vi "ADI_IMU_ADIS16448_AHRS_Madgwick2020.vi"(6 "Yaw Axis":enum16{"X", "Y", "Z"}(ring)=enum."Z", 8 "Reset?":bool, 9 "delta t":dbl, 11 "Data 2":T1) -> (3 "Output":cluster{"Pitch":dbl, "Roll":dbl, "Yaw":dbl})   [LabVIEW 2019]
panel:
  out "Quaternion":dbl[](array[numeric])
  in  "Beta":dbl=0.4
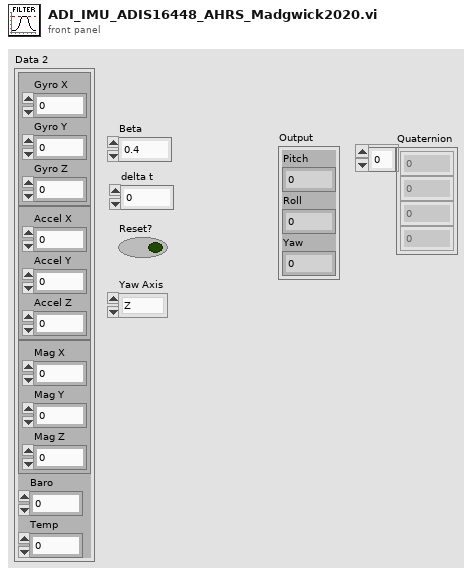
[diagram p1: front panel]
types:
  T1 = cluster{cluster{"Gyro X":dbl, "Gyro Y":dbl, "Gyro Z":dbl}, cluster{"Accel X":dbl, "Accel Y":dbl, "Accel Z":dbl}, cluster{"Mag X":dbl, "Mag Y":dbl, "Mag Z":dbl}, "Baro":dbl, "Temp":dbl}
  T2 = cluster{"Gyro X":dbl, "Gyro Y":dbl, "Gyro Z":dbl}
  T3 = cluster{"Accel X":dbl, "Accel Y":dbl, "Accel Z":dbl}
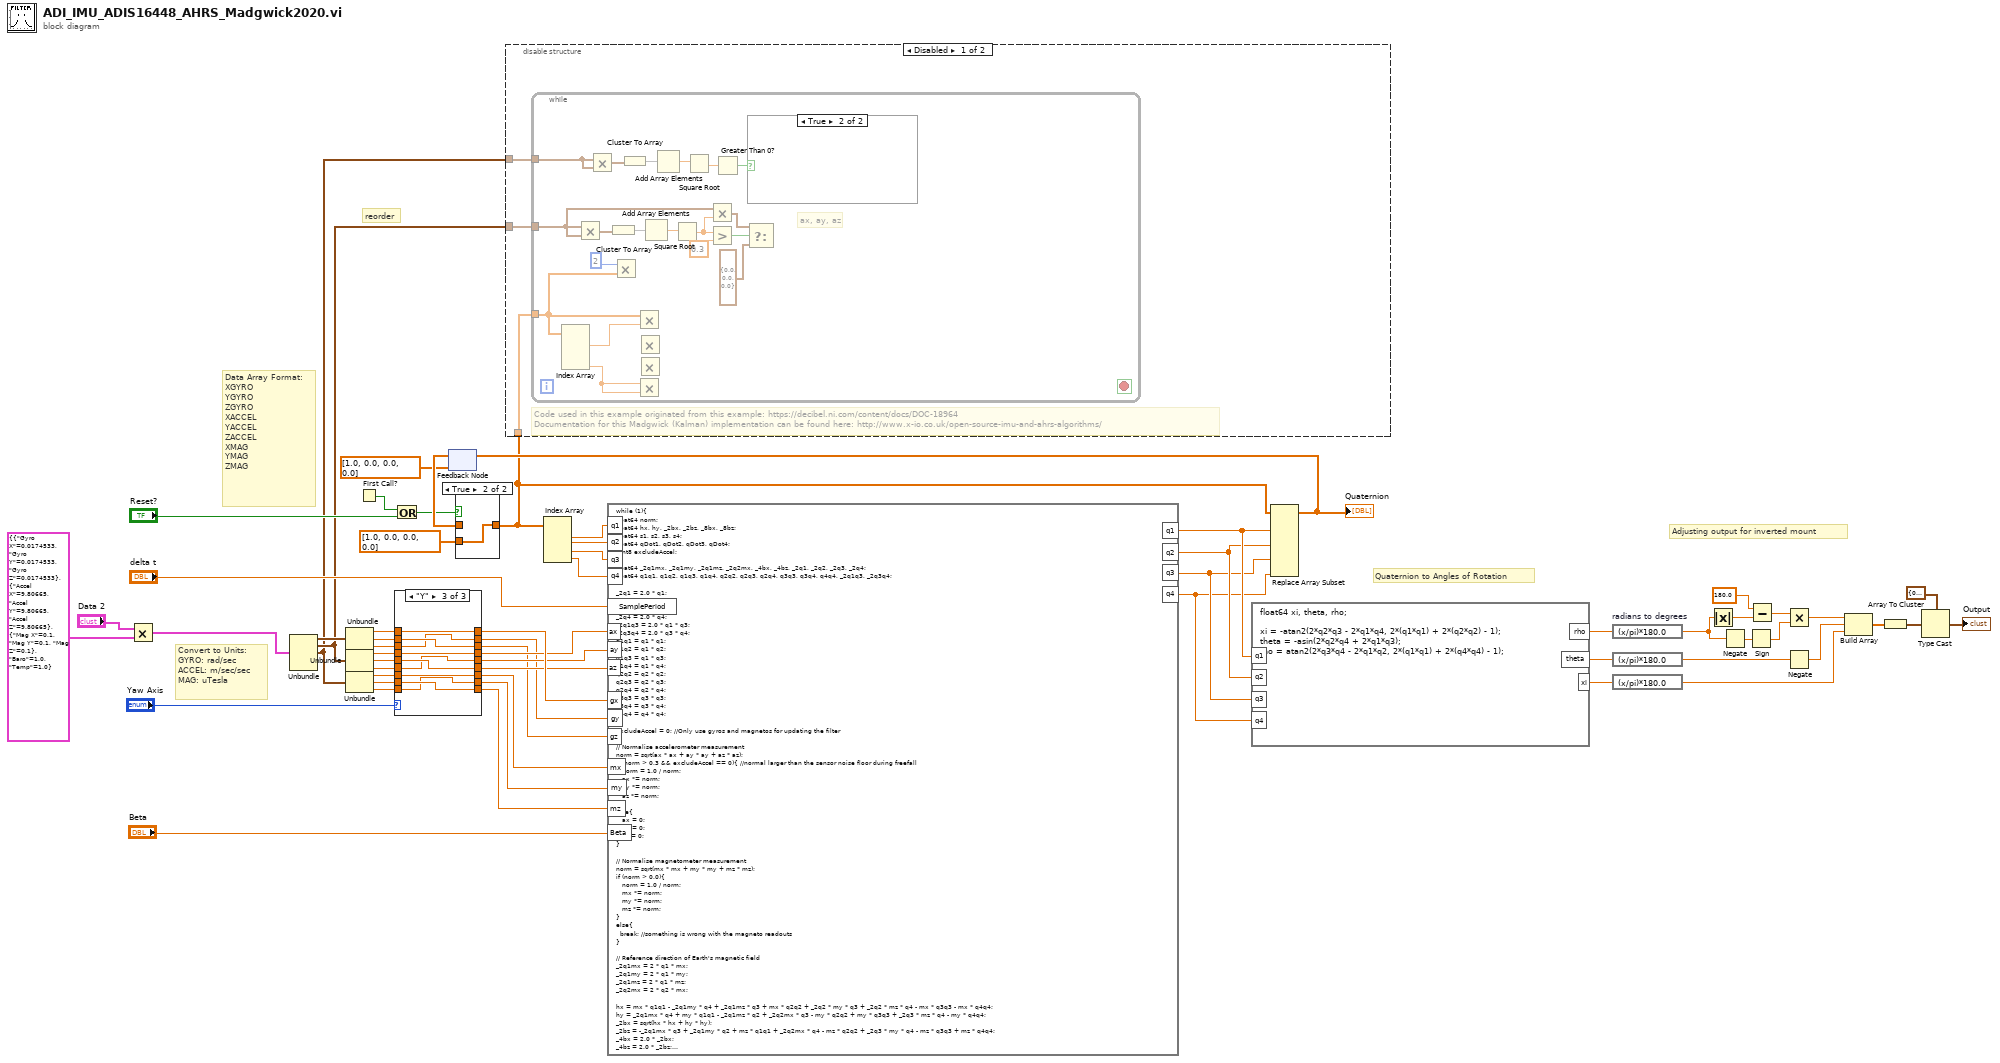
[diagram p0: block diagram]
diagram:
  # "reorder"
  # "Quaternion to Angles of Rotation"
  # "Convert to Units:\nGYRO: rad/sec\nACCEL: m/sec/sec\nMAG: uTesla"
  # "Data Array Format:\nXGYRO\nYGYRO\nZGYRO\nXACCEL\nYACCEL\nZACCEL\nXMAG\nYMAG\nZMAG"
  # "Adjusting output for inverted mount"
  n1 = Multiply(x="Data 2", y=T1 {{"Gyro X"=0.0174533, "Gyro Y"=0.0174533, "Gyro Z"=0.0174533}, {"Accel X"=9.80665, "Accel Y"=9.80665, "Accel Z"=9.80665}, {"Mag X"=0.1, "Mag Y"=0.1, "Mag Z"=0.1}, "Baro"=1.0, "Temp"=1.0} ("Data 2")) -> (x*y=w19:T1)
  n2 = Unbundle(w19) -> (w20:T2, w2:T3, w1:cluster{"Mag X":dbl, "Mag Y":dbl, "Mag Z":dbl})  [unwired: 2 out]
  n3 = Unbundle(w20) -> ("Gyro X"=w18:dbl, "Gyro Y"=w17:dbl, "Gyro Z"=w16:dbl)
  n4 = Unbundle(w2) -> ("Accel X"=w15:dbl, "Accel Y"=w14:dbl, "Accel Z"=w13:dbl)
  n5 = Unbundle(w1) -> ("Mag X"=w12:dbl, "Mag Y"=w11:dbl, "Mag Z"=w10:dbl)
  n6 = First Call?() -> (First Call?: T/F=w47:bool)
  n7 = Or(x=w47, y="Reset?") -> (x .or. y?=w48:bool)
  n8 = case shown="\"Y\"" "Yaw Axis" {
    tunnel: [w69 w78 w87] -> w60
    tunnel: [w64 w75 w84] -> w59
    tunnel: [w61 w72 w81] -> w41
    tunnel: [w65 w74 w82] -> w40
    tunnel: [w66 w73 w83] -> w39
    tunnel: [w68 w77 w85] -> w38
    tunnel: [w67 w76 w86] -> w37
    tunnel: [w62 w71 w79] -> w36
    tunnel: [w63 w70 w80] -> w35
    tunnel: w18 -> [w67 w78 w87]
    tunnel: w17 -> [w68 w77 w86]
    tunnel: w16 -> [w69 w76 w85]
    tunnel: w15 -> [w66 w75 w84]
    tunnel: w14 -> [w65 w74 w83]
    tunnel: w13 -> [w64 w73 w82]
    tunnel: w12 -> [w63 w72 w81]
    tunnel: w11 -> [w62 w71 w80]
    tunnel: w10 -> [w61 w70 w79]
    frame "X" {
    }
    frame "Z", Default {
    }
    frame "Y" {
    }
  }
  n9 = feedback #1(dbl[] [1.0, 0.0, 0.0, 0.0]) -> (w49:dbl[])
  n10 = case shown="True" w48 {
    tunnel: w49 -> [w88 _]
    tunnel: [w88 w89] -> w3
    tunnel: dbl[] [1.0, 0.0, 0.0, 0.0] -> [_ w89]
    frame False {
    }
    frame True {
    }
  }
  n11 = disable-structure shown="Disabled" {
    disable-tunnel: w3 -> [w92 _]
    disable-tunnel: w2 -> [w91 _]
    disable-tunnel: w1 -> [w90 _]
    frame Disabled {
      # "Code used in this example originated from this example: https://decibel.ni.com/content/docs/DOC-18964\nDocumentation for this Madgwick (Kalman) implementation can be found here: http://www.x-io.co.uk/open-source-imu-and-ahrs-algorithms/"
      n12 = while {
        tunnel: w92 -> [w110]
        tunnel: w91 -> [w102]
        tunnel: w90 -> [w95]
        stop <- _ stop-if-true
        # "ax, ay, az"
        n13 = Index Array(array=w110) -> (element #1=w111:dbl, element #4=w109:dbl)  [unwired: 4 in, 2 out]
        n14 = Multiply(x=w102, y=w102) -> (x*y=w108:T3)
        n15 = Multiply(x=w95, y=w95) -> (x*y=w96:cluster{"Mag X":dbl, "Mag Y":dbl, "Mag Z":dbl})
        n16 = Cluster To Array(cluster=w108) -> (array=w107:dbl[])
        n17 = Multiply(x=2 ("element"), y=w110) -> ()  [unwired: 1 out]
        n18 = Cluster To Array(cluster=w96) -> (array=w97:dbl[])
        n19 = Multiply(x=w110, y=w111) -> ()  [unwired: 1 out]
        n20 = Multiply(x=w109, y=w109) -> ()  [unwired: 1 out]
        n21 = Multiply() -> ()  [unwired: 2 in, 1 out]
        n22 = Multiply() -> ()  [unwired: 2 in, 1 out]
        n23 = Add Array Elements(numeric array=w107) -> (sum=w106:dbl)
        n24 = Add Array Elements(numeric array=w97) -> (sum=w98:dbl)
        n25 = Square Root(x=w106) -> (sqrt(x)=w103:dbl)
        n26 = Square Root(x=w98) -> (sqrt(x)=w93:dbl)
        n27 = Multiply(x=w102, y=w103) -> (x*y=w101:T3)
        n28 = Greater?(x=w103, y=0.3 ("element")) -> (0:w104:bool)
        n29 = Greater Than 0?(x=w93) -> (x > 0?=w94:bool)
        n30 = Select(t=w101, s=w104, f=T3 {"Accel X"=0.0, "Accel Y"=0.0, "Accel Z"=0.0} ("x*y")) -> (s? t:f=w99:T3)
        n31 = case shown="True" w94 {
          frame False {
          }
          frame True {
          }
        }
      }
    }
    frame Enabled {
    }
  }
  n32 = Index Array(array=w3) -> (element #1=w57:dbl, element #2=w56:dbl, element #3=w55:dbl, element #4=w54:dbl)  [unwired: 4 in]
  n33 = formula code="while (1){\nfloat64 norm;\nfloat64 hx, hy, _2bx, _2bz, _8bx, _8bz;\nfloat64 s1, s2, s3, s4;\nfloat64 qDot1, qDot2, qDot3, qDot4;\nuInt8 excludeAccel;\n\nfloat64 _2q1mx, _2q1my, _2q1mz, _2q2mx, _4bx, _4bz, _2q1, _2q2, _2q3, _2q4;\nfloat64 q1q1, q1q2, q1q3, q1q4, q2q2, q2q3, q2q4, q3q3, q3q4, q4q4, _2q1q3, _2q3q4;\n\n_2q1 = 2.0 * q1;\n_2q2 = 2.0 * q2;\n_2q3 = 2.0 * q3;\n_2q4 = 2.0 * q4;\n_2q1q3 = 2.0 * q1 * q3;\n_2q3q4 = 2.0 * q3 * q4;\nq1q1 = q1 * q1;\nq1q2 = q1 * q2;\nq1q3 = q1 * q3;\nq1q4 = q1 * q4;\nq2q2 = q2 * q2;\nq2q3 = q2 * q3;\nq2q4 = q2 * q4;\nq3q3 = q3 * q3;\nq3q4 = q3 * q4;\nq4q4 = q4 * q4;\n\nexcludeAccel = 0; //Only use gyros and magnetos for updating the filter\n\n// Normalise accelerometer measurement\nnorm = sqrt(ax * ax + ay * ay + az * az);\nif (norm > 0.3 && excludeAccel == 0){ //normal larger than the sensor noise floor during freefall\n   norm = 1.0 / norm; \n   ax *= norm;\n   ay *= norm;\n   az *= norm;\n}\nelse{\n   ax = 0;\n   ay = 0;\n   az = 0;\n}\n\n// Normalise magnetometer measurement\nnorm = sqrt(mx * mx + my * my + mz * mz);\nif (norm > 0.0){\n   norm = 1.0 / norm;\n   mx *= norm;\n   my *= norm;\n   mz *= norm;\n}\nelse{\n  break; //something is wrong with the magneto readouts\n}\n\n// Reference direction of Earth's magnetic field\n_2q1mx = 2 * q1 * mx;\n_2q1my = 2 * q1 * my;\n_2q1mz = 2 * q1 * mz;\n_2q2mx = 2 * q2 * mx;\n\nhx = mx * q1q1 - _2q1my * q4 + _2q1mz * q3 + mx * q2q2 + _2q2 * my * q3 + _2q2 * mz * q4 - mx * q3q3 - mx * q4q4;\nhy = _2q1mx * q4 + my * q1q1 - _2q1mz * q2 + _2q2mx * q3 - my * q2q2 + my * q3q3 + _2q3 * mz * q4 - my * q4q4;\n_2bx = sqrt(hx * hx + hy * hy);\n_2bz = -_2q1mx * q3 + _2q1my * q2 + mz * q1q1 + _2q2mx * q4 - mz * q2q2 + _2q3 * my * q4 - mz * q3q3 + mz * q4q4;\n_4bx = 2.0 * _2bx;\n_4bz = 2.0 * _2bz;\n_8bx = 2.0 * _4bx;\n_8bz = 2.0 * _4bz;\n\n// Gradient descent algorithm corrective step\ns1 = -_2q3 * (2.0 * q2q4 - _2q1q3 - ax) + _2q2 * (2.0 * q1q2 + _2q3q4 - ay) - _4bz * q3 * (_4bx * (0.5 - q3q3 - q4q4) + _4bz * (q2q4 - q1q3) - mx) + (-_4bx * q4 + _4bz * q2) * (_4bx * (q2q3 - q1q4) + _4bz * (q1q2 + q3q4) - my) + _4bx * q3 * (_4bx * (q1q3 + q2q4) + _4bz * (0.5 - q2q2 - q3q3) - mz);\ns2 = _2q4 * (2.0 * q2q4 - _2q1q3 - ax) + _2q1 * (2.0 * q1q2 + _2q3q4 - ay) - 4.0 * q2 * (1.0 - 2.0 * q2q2 - 2.0 * q3q3 - az) + _4bz * q4 * (_4bx * (0.5 - q3q3 - q4q4) + _4bz * (q2q4 - q1q3) - mx) + (_4bx * q3 + _4bz * q1) * (_4bx * (q2q3 - q1q4) + _4bz * (q1q2 + q3q4) - my) + (_4bx * q4 - _8bz * q2) * (_4bx * (q1q3 + q2q4) + _4bz * (0.5 - q2q2 - q3q3) - mz);\ns3 = -_2q1 * (2.0 * q2q4 - _2q1q3 - ax) + _2q4 * (2.0 * q1q2 + _2q3q4 - ay) - 4.0 * q3 * (1.0 - 2.0 * q2q2 - 2.0 * q3q3 - az) + (-_8bx * q3 - _4bz * q1) * (_4bx * (0.5 - q3q3 - q4q4) + _4bz * (q2q4 - q1q3) - mx) + (_4bx * q2 + _4bz * q4) * (_4bx * (q2q3 - q1q4) + _4bz * (q1q2 + q3q4) - my) + (_4bx * q1 - _8bz * q3) * (_4bx * (q1q3 + q2q4) + _4bz * (0.5 - q2q2 - q3q3) - mz);\ns4 = _2q2 * (2.0 * q2q4 - _2q1q3 - ax) + _2q3 * (2.0 * q1q2 + _2q3q4 - ay) + (-_8bx * q4 + _4bz * q2) * (_4bx * (0.5 - q3q3 - q4q4) + _4bz * (q2q4 - q1q3) - mx) + (-_4bx * q1 + _4bz * q3) * (_4bx * (q2q3 - q1q4) + _4bz * (q1q2 + q3q4) - my) + _4bx * q2 * (_4bx * (q1q3 + q2q4) + _4bz * (0.5 - q2q2 - q3q3) - mz);\n\nnorm = sqrt(s1 * s1 + s2 * s2 + s3 * s3 + s4 * s4);\nif (norm > 0.0){\n   norm = 1.0 / norm;  //normalise gradient step\n   s1 *= norm;\n   s2 *= norm;\n   s3 *= norm;\n   s4 *= norm;\n}\nelse{\n   break;\n}\n\n// Compute rate of change of quaternion\nqDot1 = 0.5 * (-q2 * gx - q3 * gy - q4 * gz) - Beta * s1;\nqDot2 = 0.5 * (q1 * gx + q3 * gz - q4 * gy) - Beta * s2;\nqDot3 = 0.5 * (q1 * gy - q2 * gz + q4 * gx) - Beta * s3;\nqDot4 = 0.5 * (q1 * gz + q2 * gy - q3 * gx) - Beta * s4;\n\n// Integrate to yield quaternion\nq1 += qDot1 * SamplePeriod;\nq2 += qDot2 * SamplePeriod;\nq3 += qDot3 * SamplePeriod;\nq4 += qDot4 * SamplePeriod;\n\nnorm = sqrt(q1 * q1 + q2 * q2 + q3 * q3 + q4 * q4);\nif (norm > 0.0){\n   norm = 1.0 / norm;  //normalise quaternion\n   q1 = q1 * norm;\n   q2 = q2 * norm;\n   q3 = q3 * norm;\n   q4 = q4 * norm;\n}\nbreak;\n}"("q1"=w57, "gx"=w60, "gy"=w38, "gz"=w37, "ax"=w59, "ay"=w40, "az"=w39, "mx"=w41, "my"=w36, "mz"=w35, "SamplePeriod"="delta t", "Beta"="Beta", "q2"=w56, "q3"=w55, "q4"=w54) -> ("q1"=w53:dbl, "q2"=w52:dbl, "q3"=w51:dbl, "q4"=w50:dbl)
  n34 = formula code="float64 xi, theta, rho;\n\nxi = -atan2(2*q2*q3 - 2*q1*q4, 2*(q1*q1) + 2*(q2*q2) - 1);\ntheta = -asin(2*q2*q4 + 2*q1*q3);\nrho = atan2(2*q3*q4 - 2*q1*q2, 2*(q1*q1) + 2*(q4*q4) - 1);"("q1"=w53, "q2"=w52, "q3"=w51, "q4"=w50) -> ("xi"=w43:dbl, "theta"=w45:dbl, "rho"=w44:dbl)
  n35 = Replace Array Subset(array=w3, new element #1=w53, new element #2=w52, new element #3=w51, new element #4=w50) -> (w23:dbl[])  [unwired: 4 in]
  "Quaternion" <- w23
  n36 = feedback-in #1(w23) -> ()
  n37 = expression code="(x/pi)*180.0" "radians to degrees"(w44) -> (w5:dbl)
  n38 = expression code="(x/pi)*180.0" ("radians to degrees")(w45) -> (w31:dbl)
  n39 = expression code="(x/pi)*180.0" ("radians to degrees")(w43) -> (w42:dbl)
  n40 = Absolute Value(x=w5) -> (abs(x)=w34:dbl)
  n41 = Negate(x=w5) -> (-x=w6:dbl)
  n42 = Sign(1:w6) -> (0:w4:dbl)
  n43 = Subtract(x=180.0 ("y"), y=w34) -> (x-y=w32:dbl)
  n44 = Multiply(x=w32, y=w4) -> (x*y=w29:dbl)
  n45 = Negate(x=w31) -> (-x=w30:dbl)
  n46 = Build Array(w29, w30, w42) -> (w25:dbl[])
  n47 = Array To Cluster(array=w25) -> (cluster=w26:cluster{"[0]":dbl, "[1]":dbl, "[2]":dbl})
  n48 = Type Cast(type=cluster{"Pitch":dbl, "Roll":dbl, "Yaw":dbl} {"Pitch"=0.0, "Roll"=0.0, "Yaw"=0.0} ("IMU AHRS"), x=w26) -> (*(type *) &x=→"Output":cluster{"Pitch":dbl, "Roll":dbl, "Yaw":dbl})
